vi "ROI entry-Offset Standalone.vi"() -> ()   [LabVIEW 2020]
uses:
  Typedefs/ROI move mode.ctl
  Typedefs/ROI move buttons.ctl
panel:
  in  "Step size (µm)":u8(slide)=1 min=1 max=100 step=1 scale=1.0..30.0
  in  "ROI offset arrows":T1
  in  "ROI move mode":T2
  # "ROI Offset"
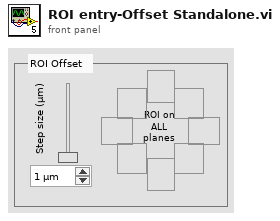
[diagram p1: front panel]
types:
  T1 = typedef "ROI move buttons.ctl" = cluster{"Right":bool, "Left":bool, "Up":bool, "Down":bool, "Up-left":bool, "Up-right":bool, "Down-left":bool, "Down-right":bool}
  T2 = typedef "ROI move mode.ctl" = enum16{"ROI on ALL planes", "ROI on current plane"}
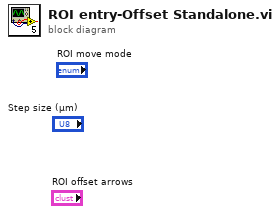
[diagram p0: block diagram]
diagram:
